vi "execute_lua_script.vi"(4 "nresults":i32, 6 "nargs":i32, 8 "error in (no error)":errorcluster, 10 "lua script":string, 11 "Lua in":refnum<class "Lua.lvclass">) -> (0 "error out":errorcluster, 3 "Lua out":refnum<class "Lua.lvclass">)   [LabVIEW 2020, in "Lua for LabVIEW.lvlib" / "Lua.lvclass"]
doc: "Load and execute a Lua script. Specify the number of return values expected from the script using the nresults argument. For example, to return a number from a script, the script could end with:\n\n...\nreturn my_number_result\n\nIf nargs = -1, then any values on the stack at the time of the call will be passed to the script.\nIf nresult = -1, then all values returned from the script will be left on the stack after the call."
uses:
  Lua.lvclass
  Lua.lvclass/Lua.ctl
  lib/lua.dll/types/lua_error_code_offset.vi
  lib/lua.dll/lua_type.vi
  lib/lua.dll/luaL_typename.vi
  lib/lua.dll/lua_tostring.vi
  lib/lua.dll/lua_toboolean.vi
  lib/lua.dll/lua_tonumber.vi
  lib/lua.dll/lua_tolstring.vi
  lib/lua.dll/lua_pop.vi
  lib/lua.dll/lua_typename.vi
  lib/lua.dll/lua_settop.vi
  <vilib>/Utility/error.llb/Error Cluster From Error Code.vi
  lib/lua.dll/lua.dll.lvlib
panel:
  out "stack":string[](array[string])
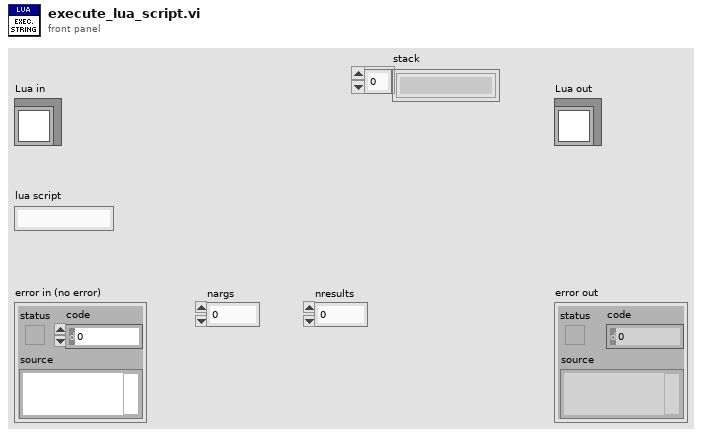
[diagram p1: front panel]
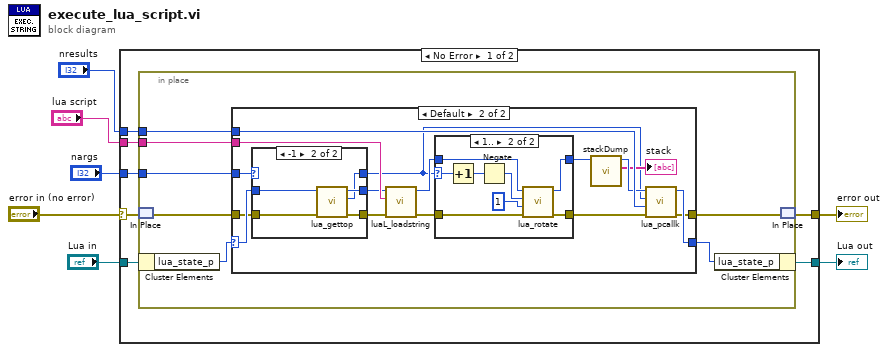
[diagram p0: block diagram]
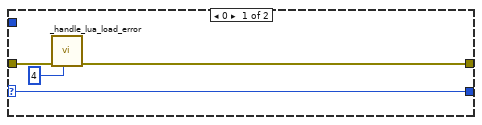
[diagram p2: hidden frame]
diagram:
  n1 = case shown="No Error" "error in (no error)" {
    selector: "error in (no error)" -> [w11 w61]
    tunnel: [w12 w61] -> w4
    tunnel: [w13 w60] -> w7
    tunnel: "Lua in" -> [w14 w60]
    tunnel: "nargs" -> [w10 _]
    tunnel: "nresults" -> [w9 _]
    tunnel: "lua script" -> [w8 _]
    frame No Error {
      n2 = in-place {
        in-place-border: w10 -> [w17]
        in-place-border: w9 -> [w16]
        in-place-border: w8 -> [w15]
        n3 = in-place-match #1(w11) -> (w19:errorcluster)
        n4 = in-place-cluster #2(w14) -> ("lua_state_p"=w20:u64)
        n5 = case shown="Default" w20 {
          selector: w20 -> [w25 w29]
          tunnel: [w25 w41] -> w21
          tunnel: w19 -> [w22 w26]
          tunnel: [w23 w39] -> w18
          tunnel: w17 -> [_ w31]
          tunnel: w16 -> [_ w40]
          tunnel: w15 -> [_ w36]
          frame 0 {
            n6 = call "_handle_lua_load_error.vi"("lua_load errcode"=4, "error in (no error)"=w22) -> ("error out"=w23:errorcluster)  [unwired: 9 in]
          }
          frame Default {
            n7 = case shown="-1" w31 {
              selector: w31 -> [w44 _]
              tunnel: [w44 w47] -> w30
              tunnel: w29 -> [w42 w49]
              tunnel: [w42 w48] -> w28
              tunnel: [w43 w46] -> w27
              tunnel: w26 -> [w43 w45]
              frame Default {
              }
              frame -1 {
                n8 = call "lua_gettop.vi"("error in (no error)"=w45, "lua_state_p"=w49) -> ("error out"=w46:errorcluster, "index"=w47:i32, "lua_state_p out"=w48:u64)  [unwired: 7 in]
              }
            }
            n9 = call "luaL_loadstring.vi"("error in (no error)"=w27, "lua chunk"=w36, "lua_state_p"=w28) -> ("error out"=w38:errorcluster, "lua_state_p out"=w37:u64)  [unwired: 7 in]
            n10 = case shown="1.." w30 {
              selector: w30 -> [_ w53]
              tunnel: w37 -> [w51 w59]
              tunnel: [w51 w58] -> w34
              tunnel: [w50 w57] -> w35
              tunnel: w38 -> [w50 w56]
              frame Default {
              }
              frame 1.. {
                n11 = Increment(x=w53) -> (x+1=w52:i32)
                n12 = Negate(x=w52) -> (-x=w55:i32)
                n13 = call "lua_rotate.vi"("error in (no error)"=w56, "n"=1, "index"=w55, "lua_state_p"=w59) -> ("error out"=w57:errorcluster, "lua_state_p out"=w58:u64)  [unwired: 6 in]
              }
            }
            n14 = call "stackDump.vi"("lua_state_p"=w34) -> ("stack"=→"stack":string[], "lua_state_p out"=w33:u64)  [unwired: 8 in, 1 out]
            n15 = call "lua_pcallk.vi"("error in (no error)"=w35, "nresults"=w40, "nargs"=w30, "lua_state_p"=w33) -> ("error out"=w39:errorcluster, "lua_state_p out"=w41:u64)  [unwired: 6 in]
          }
        }
        n16 = in-place-cluster #2("lua_state_p"=w21) -> (w13:refnum<class "Lua.lvclass">)
        n17 = in-place-match #1(w18) -> (w12:errorcluster)
      }
    }
    frame Error {
    }
  }
  "error out" <- w4
  "Lua out" <- w7
